vi "Config Aout Bound.vi"(0 "VISA resource name":refnum<visa-resource-name>, 1 "Upper Capacitance (10.0 V)":dbl=10.0 min=-160.0 max=160.0 format="%#_6f", 2 "Upper Loss (10.0 V)":dbl=10.0 min=-160.0 max=160.0 format="%#_6f", 3 "Lower Capacitance (-10.0 V)":dbl=-10.0 min=-160.0 max=160.0 format="%#_6f", 4 "Lower Loss (-10.0 V)":dbl=-10.0 min=-160.0 max=160.0 format="%#_6f", 5 "error in":errorcluster) -> (14 "VISA resource name out":refnum<visa-resource-name>, 19 "error out":errorcluster)   [LabVIEW 2019, in "Andeen-Hagerling 2700(400 firmware).lvlib"]
doc: "Sets the upper and lower bounds of the capacitance and loss channel output voltages in volts."
uses:
  Andeen-Hagerling 2700(400 firmware).lvlib
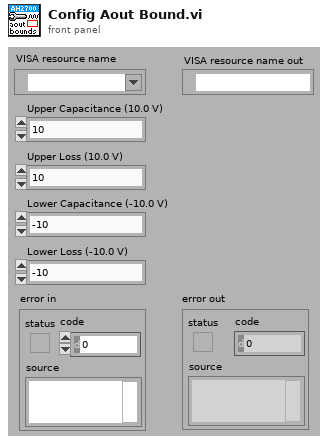
[diagram p1: front panel]
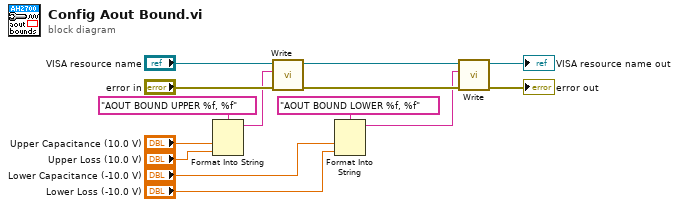
[diagram p0: block diagram]
diagram:
  n1 = Format Into String(format string="AOUT BOUND UPPER %f, %f", "Upper Capacitance (10.0 V)", "Upper Loss (10.0 V)") -> (resulting string=w9:string)  [unwired: 2 in, 1 out]
  n2 = call "Write.vi"("error in"="error in", "command"=w9, "VISA resource name"="VISA resource name") -> ("error out"=w6:errorcluster, "VISA resource name out"=w8:refnum<visa-resource-name>)  [unwired: 7 in]
  n3 = Format Into String(format string="AOUT BOUND LOWER %f, %f", "Lower Capacitance (-10.0 V)", "Lower Loss (-10.0 V)") -> (resulting string=w2:string)  [unwired: 2 in, 1 out]
  n4 = call "Write.vi"("error in"=w6, "command"=w2, "VISA resource name"=w8) -> ("error out"=→"error out":errorcluster, "VISA resource name out"=→"VISA resource name out":refnum<visa-resource-name>)  [unwired: 7 in]
